vi "_prepare_measure.vi"(8 "error in (no error)":errorcluster, 11 "UV-VIS_AVANTES in":refnum<class "UV-VIS_AVANTES.lvclass">) -> (0 "error out":errorcluster, 2 "return type":i32, 3 "UV-VIS_AVANTES out":refnum<class "UV-VIS_AVANTES.lvclass">)   [LabVIEW 2020, in "UV-VIS_AVANTES.lvclass"]
uses:
  UV-VIS_AVANTES.lvclass
  C:/dev/TRANCON/Classes/Detector/Detector.lvclass
  def_measure_parameters.ctl
  Detector.lvclass/Detector.ctl
  UV-VIS_AVANTES.lvclass/UV-VIS_AVANTES.ctl
  Detector.lvclass
panel:
  in  "MeasConfigType":T1
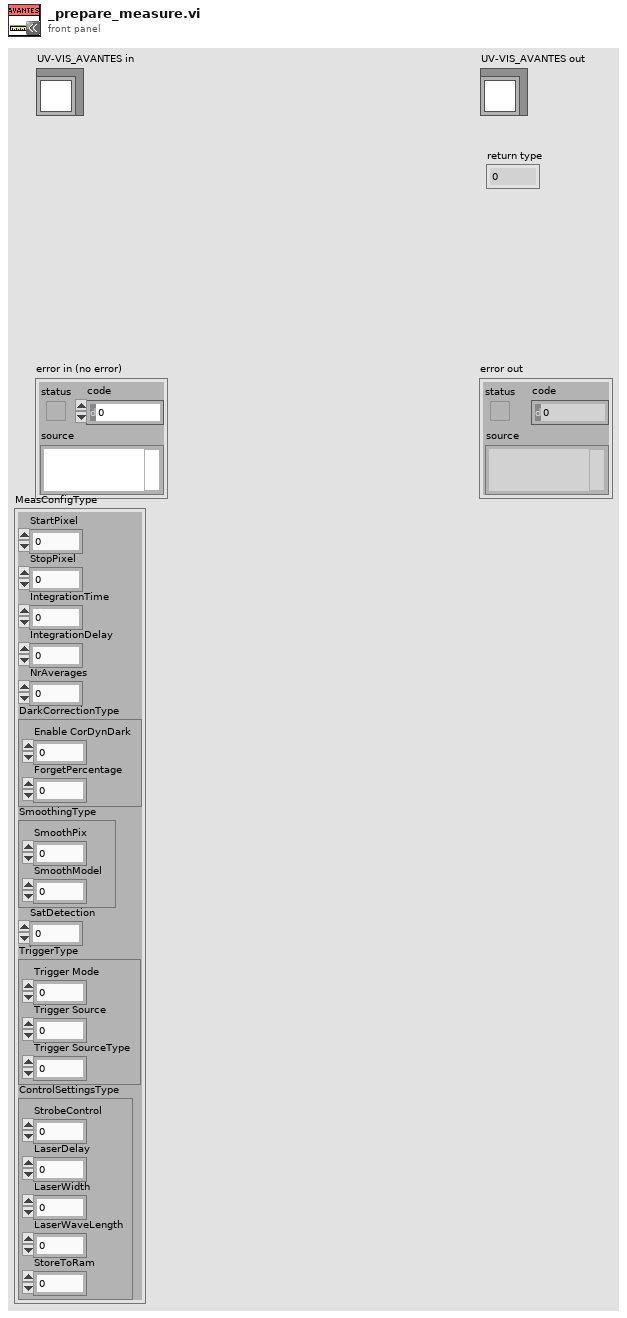
[diagram p1: front panel]
types:
  T1 = typedef "UV-VIS_AVANTES.lvclass/def_measure_parameters.ctl" = cluster{"StartPixel":u16, "StopPixel":u16, "IntegrationTime":sgl, "IntegrationDelay":u32, "NrAverages":u32, "DarkCorrectionType":cluster{"Enable CorDynDark":u8, "ForgetPercentage":u8}, "SmoothingType":cluster{"SmoothPix":u16, "SmoothModel":u8}, "SatDetection":u8, "TriggerType":cluster{"Trigger Mode":u8, "Trigger Source":u8, "Trigger SourceType":u8}, "ControlSettingsType":cluster{"StrobeControl":u16, "LaserDelay":u32, "LaserWidth":u32, "LaserWaveLength":sgl, "StoreToRam":u16}}
  T2 = typedef "UV-VIS_AVANTES.lvclass/def_parameters.ctl" = cluster{"Len":u16, "ConfigVersion":u16, "UserFriendlyId":u8[], "DetectorType":cluster{"SensorType":u8, "NrPixels":u16, "Fit":sgl[], "NLEnable":u8, "NLCorrect":dbl[], "LowNLCounts":dbl, "HighNLCounts":dbl, "Gain":sgl[], "Reserved":sgl, "Offset":sgl[], "Extern Offset":sgl, "DefectivePixels":u16[]}, "IrradianceType":cluster{"SpectrumCalibrationType":cluster{"SmoothingType":cluster{"m_SmoothPix":u16, "SmoothModel":u8}, "CalInttime":sgl, "CalibConvers":sgl[]}, "CalibrationType":u8, "FiberDiameter":i32}, "SpectrumCalibrationType":cluster{"SmoothingType":cluster{"m_SmoothPix":u16, "SmoothModel":u8}, "CalInttime":sgl, "CalibConvers":sgl[]}, "SpectrumCorrectionType":sgl[], "StandAloneType":cluster{"StandAloneType":u8, "MeasConfigType":cluster{"StartPixel":u16, "StopPixel":u16, "IntegrationTime":sgl, "IntegrationDelay":u32, "NrAverages":u32, "DarkCorrectionType":cluster{"Enable CorDynDark":u8, "ForgetPercentage":u8}, "SmoothingType":cluster{"SmoothPix":u16, "SmoothModel":u8}, "SatDetection":u8, "TriggerType":cluster{"Trigger Mode":u8, "Trigger Source":u8, "Trigger SourceType":u8}, "ControlSettingsType":cluster{"StrobeControl":u16, "LaserDelay":u32, "LaserWidth":u32, "LaserWaveLength":sgl, "StoreToRam":u16}}, "Nmsr":i16}, "DynamicStorageType":cluster{"Nmsr":i32, "Reserved":u8[]}, "TempSensorType":sgl[], "TecControlType":cluster{"Enable":u8, "Setpoint":sgl, "Fit[NR_DAC_POL_COEF]":sgl[]}, "ProcessControlType":cluster{"AnalogLow":sgl[], "AnalogHigh":sgl[], "DigitalLow":sgl[], "DigitalHigh":sgl[]}, "EthernetSettingsType":cluster{"IpAddr":u32, "NetMask":u32, "Gateway":u32, "DhcpEnabled":u8, "TcpPort":u16, "LinkStatus":u8}, "Reserved":u8[]}
  T3 = cluster{"Enable CorDynDark":u8, "ForgetPercentage":u8}
  T4 = cluster{"Trigger Mode":u8, "Trigger Source":u8, "Trigger SourceType":u8}
  T5 = cluster{"StrobeControl":u16, "LaserDelay":u32, "LaserWidth":u32, "LaserWaveLength":sgl, "StoreToRam":u16}
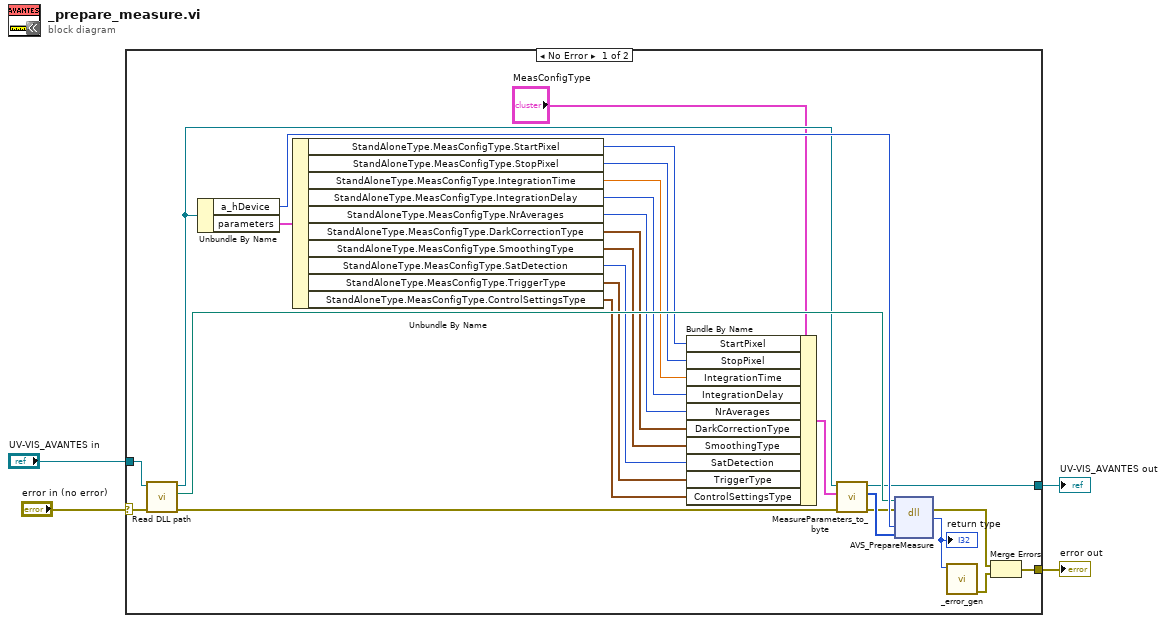
[diagram p0: block diagram]
diagram:
  n1 = case shown="No Error" "error in (no error)" {
    selector: "error in (no error)" -> [w29 w32]
    tunnel: [w7 w32] -> w3
    tunnel: [w22 w31] -> w1
    tunnel: "UV-VIS_AVANTES in" -> [w30 w31]
    frame No Error {
      n2 = call "Read DLL path.vi"("error in (no error)"=w29, "Detector in"=w30) -> ("error out"=w25:errorcluster, "DLL path"=w27:path, "Detector out"=w23:refnum<class "UV-VIS_AVANTES.lvclass">)  [unwired: 7 in]
      n3 = Unbundle By Name(w23) -> ("a_hDevice"=w28:i32, "parameters"=w21:T2)
      n4 = Unbundle By Name(w21) -> ("StandAloneType.MeasConfigType.StartPixel"=w20:u16, "StandAloneType.MeasConfigType.StopPixel"=w19:u16, "StandAloneType.MeasConfigType.IntegrationTime"=w18:sgl, "StandAloneType.MeasConfigType.IntegrationDelay"=w17:u32, "StandAloneType.MeasConfigType.NrAverages"=w16:u32, "StandAloneType.MeasConfigType.DarkCorrectionType"=w15:T3, "StandAloneType.MeasConfigType.SmoothingType"=w14:cluster{"SmoothPix":u16, "SmoothModel":u8}, "StandAloneType.MeasConfigType.SatDetection"=w13:u8, "StandAloneType.MeasConfigType.TriggerType"=w12:T4, "StandAloneType.MeasConfigType.ControlSettingsType"=w11:T5)
      n5 = Bundle By Name(cluster="MeasConfigType", "StartPixel"=w20, "StopPixel"=w19, "IntegrationTime"=w18, "IntegrationDelay"=w17, "NrAverages"=w16, "DarkCorrectionType"=w15, "SmoothingType"=w14, "SatDetection"=w13, "TriggerType"=w12, "ControlSettingsType"=w11) -> (w6:T1)
      n6 = call "MeasureParameters_to_byte.vi"("error in (no error)"=w25, "MeasConfigType"=w6, "UV-VIS_AVANTES in"=w23) -> ("error out"=w24:errorcluster, "Measure byte  array"=w26:u8[], "UV-VIS_AVANTES out"=w22:refnum<class "UV-VIS_AVANTES.lvclass">)  [unwired: 6 in]
      n7 = dll-call lib="C:/AvaSpecX64-DLL_9.4/examples/LabView/LabViewSingleChan/avaspec.dll" fn="AVS_PrepareMeasure"(path in=w27, error in=w24, "a_hDevice"=w28, "MeasConfArray"=w26) -> (error out=w8:errorcluster, "return type"=w9:i32)  [unwired: 3 in, 1 out]
      "return type" <- w9
      n8 = call "_error_gen.vi"("return type"=w9) -> ("error out"=w10:errorcluster)  [unwired: 10 in]
      n9 = Merge Errors(w8, w10) -> (w7:errorcluster)
    }
    frame Error {
    }
  }
  "error out" <- w3
  "UV-VIS_AVANTES out" <- w1
